vi "王廷瑋記憶遊戲.vi"() -> ()   [LabVIEW 2014]
panel:
  in  "難易度":enum16{"Easy", "Medium", "Hard"}(ring)
  out "Numeric":i32
  in  "?":bool
  in  "?":bool
  out "score":u8
  in  "?":T1
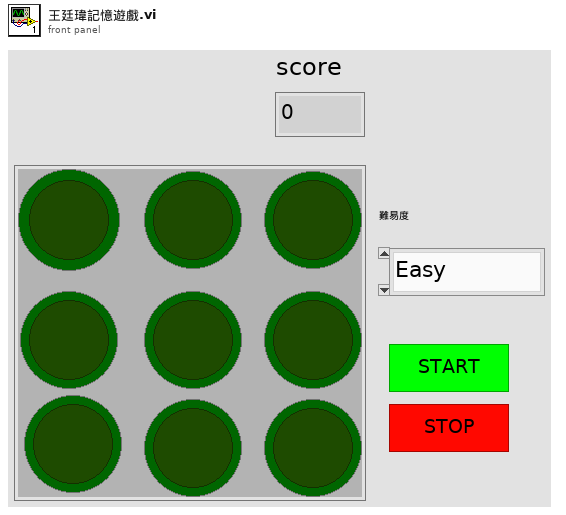
[diagram p1: front panel]
types:
  T1 = cluster{bool, bool, bool, bool, bool, bool, bool, bool, bool}
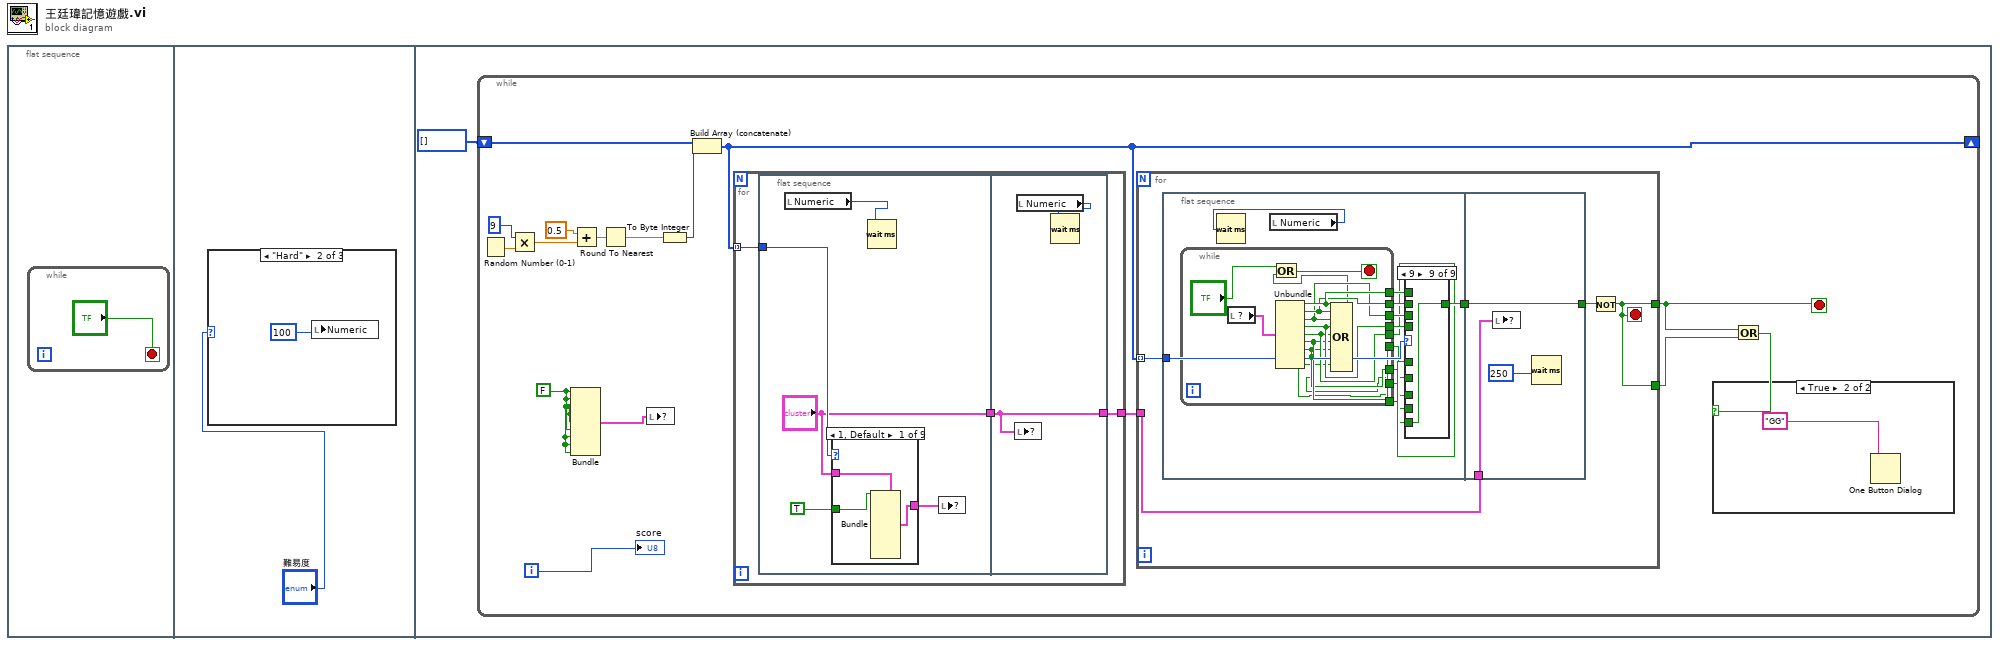
[diagram p0: block diagram]
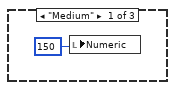
[diagram p2: hidden frame]
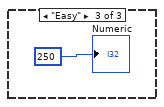
[diagram p3: hidden frame]
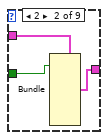
[diagram p13: hidden frame]
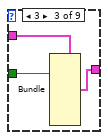
[diagram p14: hidden frame]
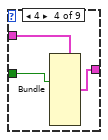
[diagram p15: hidden frame]
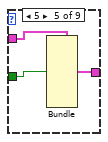
[diagram p16: hidden frame]
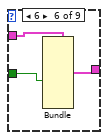
[diagram p17: hidden frame]
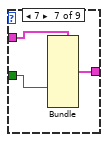
[diagram p18: hidden frame]
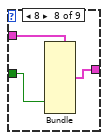
[diagram p19: hidden frame]
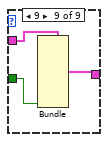
[diagram p20: hidden frame]
diagram:
  n1 = flat-sequence {
    frame #0 {
      n2 = while {
        stop <- "?" stop-if-true
      }
    }
    frame #1 {
      n3 = case shown="\"Hard\"" "難易度" {
        frame "Medium" {
          n4 = local write "Numeric"(150) -> ()
        }
        frame "Hard" {
          n5 = local write "Numeric"(100) -> ()
        }
        frame "Easy" {
          "Numeric" <- 250
        }
      }
    }
    frame #2 {
      n6 = while {
        shift-right: [w13] -> _
        shift-left: i32[] [] -> [w15]
        i -> [w14]
        stop <- w8 stop-if-true
        w7 = FALSE
        n7 = Random Number (0-1)() -> (number: 0 to 1=w22:dbl)
        n8 = Multiply(x=i8 9, y=w22) -> (x*y=w20:dbl)
        n9 = Bundle(w7, w7, w7, w7, w7, w7, w7, w7, w7) -> (w11:T1)  [unwired: 1 in]
        n10 = Add(x=0.5, y=w20) -> (x+y=w18:dbl)
        n11 = Round To Nearest(number=w18) -> (nearest integer value=w17:dbl)
        n12 = local write item#?(w11) -> ()
        n13 = To Byte Integer(number=w17) -> (8bit integer=w16:i8)
        n14 = Build Array (concatenate)(w15, w16) -> (w13:i32[])
        n15 = for {
          tunnel: w13 -> [w68] mode=indexing
          tunnel: [w66] -> w12
          n16 = flat-sequence {
            tunnel: w68 -> [w73]
            tunnel: ["?"] -> w67
            tunnel: w67 -> [w102]
            tunnel: [w102] -> w66
            frame #0 {
              n17 = local read "Numeric"() -> (w69:i32)
              n18 = case shown="1, Default" w73 {
                tunnel: "?" -> [w76 w79 w81 w85 w88 w91 w94 w97 w100]
                tunnel: TRUE -> [w75 w78 w82 w84 w87 w90 w93 w96 w99]
                tunnel: [w74 w77 w80 w83 w86 w89 w92 w95 w98] -> w71
                frame 1, Default {
                  n19 = Bundle(cluster=w76, w75) -> (w74:T1)  [unwired: 8 in]
                }
                frame 2 {
                  n20 = Bundle(cluster=w79, w78) -> (w77:T1)  [unwired: 8 in]
                }
                frame 3 {
                  n21 = Bundle(cluster=w81, w82) -> (w80:T1)  [unwired: 8 in]
                }
                frame 4 {
                  n22 = Bundle(cluster=w85, w84) -> (w83:T1)  [unwired: 8 in]
                }
                frame 5 {
                  n23 = Bundle(cluster=w88, w87) -> (w86:T1)  [unwired: 8 in]
                }
                frame 6 {
                  n24 = Bundle(cluster=w91, w90) -> (w89:T1)  [unwired: 8 in]
                }
                frame 7 {
                  n25 = Bundle(cluster=w94, w93) -> (w92:T1)  [unwired: 8 in]
                }
                frame 8 {
                  n26 = Bundle(cluster=w97, w96) -> (w95:T1)  [unwired: 8 in]
                }
                frame 9 {
                  n27 = Bundle(cluster=w100, w99) -> (w98:T1)  [unwired: 8 in]
                }
              }
              n28 = Wait (ms)(milliseconds to wait=w69) -> ()  [unwired: 1 out]
              n29 = local write item#?(w71) -> ()
            }
            frame #1 {
              n30 = local write item#?(w102) -> ()
              n31 = local read "Numeric"() -> (w101:i32)
              n32 = Wait (ms)(milliseconds to wait=w101) -> ()  [unwired: 1 out]
            }
          }
        }
        n33 = for {
          tunnel: w13 -> [w28] mode=indexing
          tunnel: [w24] -> w8
          tunnel: w12 -> [w25]
          tunnel: [w24] -> w10
          stop <- w24 stop-if-true
          n34 = flat-sequence {
            tunnel: w28 -> [w40]
            tunnel: [w35] -> w27
            tunnel: w27 -> [w64]
            tunnel: w25 -> [w65]
            tunnel: [w64] -> w26
            frame #0 {
              n35 = while {
                tunnel: [w59] -> w39
                tunnel: [w58] -> w38
                tunnel: [w57] -> w37
                tunnel: [w56] -> w36
                tunnel: [w55] -> w34
                tunnel: [w54] -> w33
                tunnel: [w53] -> w32
                tunnel: [w52] -> w31
                tunnel: [w51] -> w30
                stop <- w61 stop-if-true
                n36 = local read item#?() -> (w62:T1)
                n37 = Unbundle(w62) -> (w59:bool, w58:bool, w57:bool, w56:bool, w55:bool, w54:bool, w53:bool, w52:bool, w51:bool)
                n38 = Compound Arithmetic op=OR(w59, w58, w57, w56, w55, w54, w53, w52, w51) -> (w50:bool)
                n39 = Or(x="?", y=w50) -> (x .or. y?=w61:bool)
              }
              n40 = local read "Numeric"() -> (w29:i32)
              n41 = Wait (ms)(milliseconds to wait=w29) -> ()  [unwired: 1 out]
              n42 = case shown="9" w40 {
                tunnel: [w41 w42 w43 w44 w45 w46 w47 w48 w49] -> w35
                tunnel: w39 -> [w41 _ _ _ _ _ _ _ _]
                tunnel: w38 -> [_ w42 _ _ _ _ _ _ _]
                tunnel: w37 -> [_ _ w43 _ _ _ _ _ _]
                tunnel: w36 -> [_ _ _ w44 _ _ _ _ _]
                tunnel: w34 -> [_ _ _ _ w45 _ _ _ _]
                tunnel: w33 -> [_ _ _ _ _ w46 _ _ _]
                tunnel: w32 -> [_ _ _ _ _ _ w47 _ _]
                tunnel: w31 -> [_ _ _ _ _ _ _ w48 _]
                tunnel: w30 -> [_ _ _ _ _ _ _ _ w49]
                frame 1, Default {
                }
                frame 2 {
                }
                frame 3 {
                }
                frame 4 {
                }
                frame 5 {
                }
                frame 6 {
                }
                frame 7 {
                }
                frame 8 {
                }
                frame 9 {
                }
              }
            }
            frame #1 {
              n43 = local write item#?(w65) -> ()
              n44 = Wait (ms)(milliseconds to wait=250) -> ()  [unwired: 1 out]
            }
          }
          n45 = Not(x=w26) -> (.not. x?=w24:bool)
        }
        n46 = Or(x=w8, y=w10) -> (x .or. y?=w9:bool)
        n47 = case shown="True" w9 {
          frame False {
          }
          frame True {
            n48 = One Button Dialog(message="GG") -> ()  [unwired: 1 in, 1 out]
          }
        }
        "score" <- w14
      }
    }
  }
